vi "calculate.vi"(8 "error in (no error)":errorcluster, 10 "Numbers.lvclass":refnum<class "Numbers.lvclass">, 11 "Divide in":refnum<class "Divide.lvclass">) -> (0 "error out":errorcluster, 3 "Divide out":refnum<class "Divide.lvclass">)   [LabVIEW 2017, in "Divide.lvclass"]
uses:
  Divide.lvclass
  Numbers Class/Numbers.lvclass
  Numbers Class/Numbers.lvclass/Numbers.ctl
  ConsoleOut/Print Options.ctl
  Chain Class/Chain.lvclass
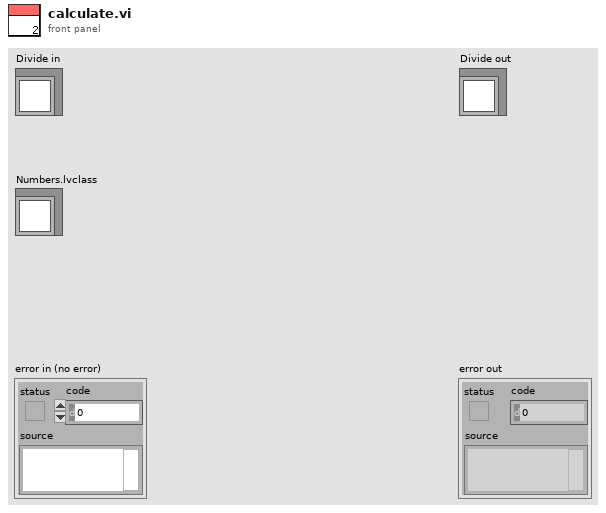
[diagram p1: front panel]
types:
  T1 = typedef "Print Options.ctl" = enum16{"Create", "Get Reference", "Print", "Print Header", "Close"}
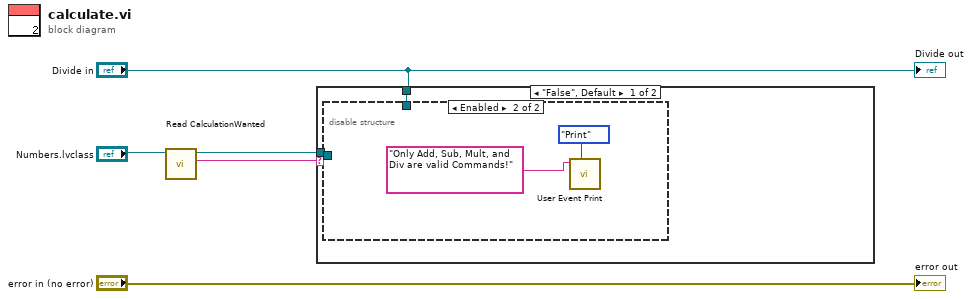
[diagram p0: block diagram]
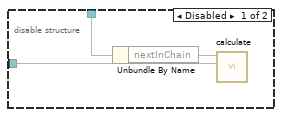
[diagram p2: hidden frame]
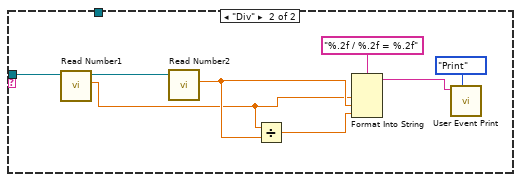
[diagram p3: hidden frame]
diagram:
  n1 = call "Read CalculationWanted.vi"("Numbers in"="Numbers.lvclass") -> ("CalculationWanted"=w4:string, "Numbers out"=w3:refnum<class "Numbers.lvclass">)  [unwired: 8 in, 1 out]
  n2 = case shown="\"False\", Default" w4 {
    tunnel: w3 -> [w7 w20]
    tunnel: "Divide in" -> [w6 _]
    frame "False", Default {
      n3 = disable-structure shown="Enabled" {
        disable-tunnel: w7 -> [w10 _]
        disable-tunnel: w6 -> [w9 _]
        frame Disabled {
          n4 = Unbundle By Name(w9) -> ("nextInChain"=w8:refnum<class "Chain.lvclass">)
          n5 = call-dynamic "calculate.vi"("Numbers.lvclass"=w10, "Chain in"=w8) -> ()  [unwired: 8 in, 2 out]
        }
        frame Enabled {
          n6 = call "User Event Print.vi"("Options"=Print_Options."Print", "String to Print"="Only Add, Sub, Mult, and Div are valid Commands!" ("message")) -> ()  [unwired: 8 in, 2 out]
        }
      }
    }
    frame "Div" {
      n7 = call "Read Number1.vi"("Numbers in"=w20) -> ("Number1"=w15:dbl, "Numbers out"=w19:refnum<class "Numbers.lvclass">)  [unwired: 8 in, 1 out]
      n8 = call "Read Number2.vi"("Numbers in"=w19) -> ("Number2"=w16:dbl)  [unwired: 8 in, 2 out]
      n9 = Divide(x=w15, y=w16) -> (x/y=w17:dbl)
      n10 = Format Into String(format string="%.2f / %.2f = %.2f", w15, w16, w17) -> (resulting string=w14:string)  [unwired: 2 in, 1 out]
      n11 = call "User Event Print.vi"("Options"=Print_Options."Print", "String to Print"=w14) -> ()  [unwired: 8 in, 2 out]
    }
  }
  "error out" <- "error in (no error)"
  "Divide out" <- "Divide in"
